vi "Actor Core.vi"(8 "error in":errorcluster, 11 "Nested in":refnum<class "User Interface.lvclass">) -> (0 "error out":errorcluster, 3 "Actor out":refnum<class "Actor.lvclass">)   [LabVIEW 2020, in "User Interface.lvlib" / "User Interface.lvclass"]
doc: "(<B>Filename</B>: Actor Framework.lvlib:Actor.lvclass:Actor Core.vi)\n\nReceives messages to the actor, reacts to them, and initiates any error handling that may shut the actor down.\n\nDescendant classes may override this VI to append parallel tasks for the actor to complete while it handles messages. Overrides use the Call Parent Method node."
uses:
  User Interface.lvclass
  <vilib>/ActorFramework/Actor/Actor.lvclass
  <vilib>/ActorFramework/Stop Msg/Stop Msg.lvclass
  Paquetes Disonibles/Paquetes Disonibles.lvclass
  Manejador de Turnos/Manejador de Turnos.lvclass
  Dinero/Dinero.lvclass
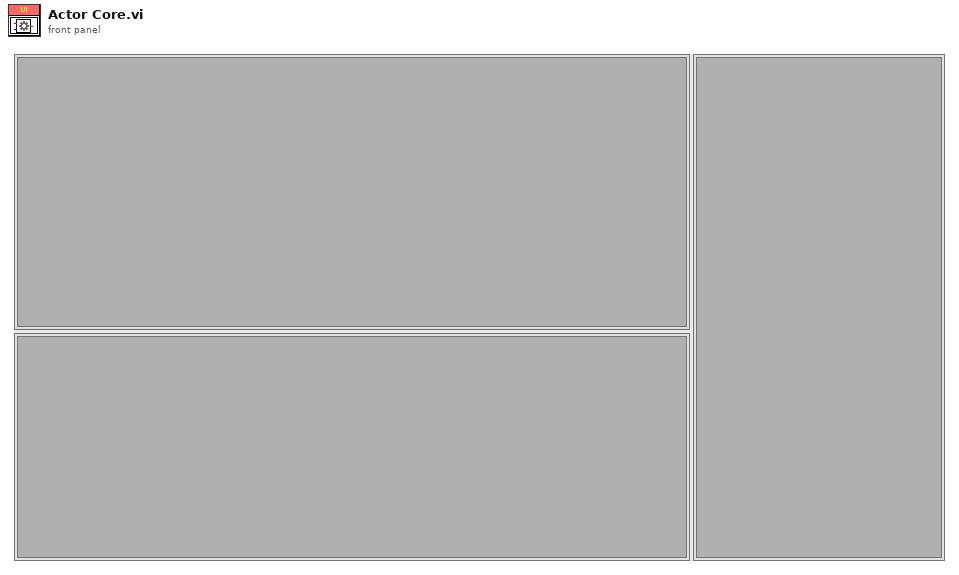
[diagram p1: front panel]
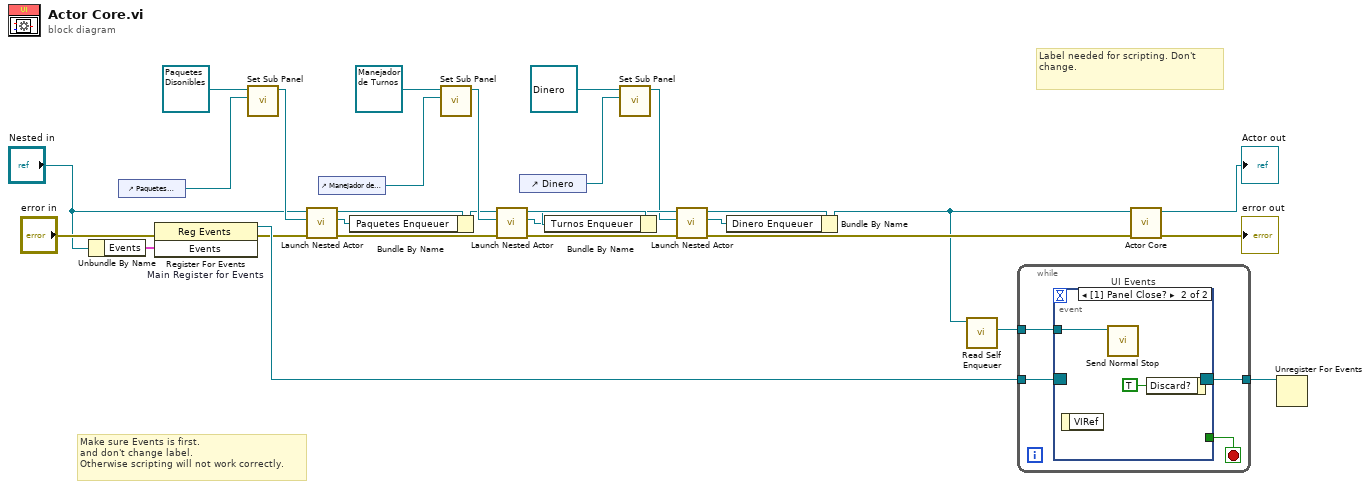
[diagram p0: block diagram]
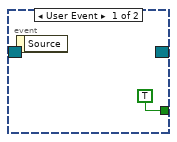
[diagram p2: hidden frame]
diagram:
  # "Label needed for scripting. Don't change."
  # "Make sure Events is first.\nand don't change label.\nOtherwise scripting will not work correctly."
  n1 = Unbundle By Name("Nested in") -> ("Events"=w27:cluster{"Stop":refnum<user-event>})
  n2 = control-ref of="Paquetes disponibles"() -> (w3:refnum<vi>)
  n3 = register-events "Main Register for Events"(error in="error in", w27) -> (reference out=w28:refnum<event-registration>, error out=w19:errorcluster)  [unwired: 1 in]
  n4 = call "Set Sub Panel.vi"("Sub Panel"=w3, "Paquetes Disonibles in"=refnum<class "Paquetes Disonibles.lvclass"> refnum ("Paquetes Disonibles.lvlib:Paquetes Disonibles.lvclass")) -> ("Paquetes Disonibles out"=w18:refnum<class "Paquetes Disonibles.lvclass">)  [unwired: 8 in, 1 out]
  n5 = call <vilib>:"Launch Nested Actor.vi"("error in (no error)"=w19, "Nested Actor"=w18, "Caller Actor in"="Nested in") -> ("error out"=w17:errorcluster, "Nested Actor's Enqueuer"=w4:refnum<class "Message Enqueuer.lvclass">, "Caller Actor out"=w20:refnum<class "User Interface.lvclass">)  [unwired: 6 in]
  n6 = control-ref of="Manejador de turnos"() -> (w2:refnum<vi>)
  n7 = Bundle By Name(cluster=w20, "Paquetes Enqueuer"=w4) -> (w5:refnum<class "User Interface.lvclass">)
  n8 = call "Set Sub Panel.vi"("Sub Panel"=w2, "Manejador de Turnos in"=refnum<class "Manejador de Turnos.lvclass"> refnum ("Manejador de Turnos.lvlib:Manejador de Turnos.lvclass")) -> ("Manejador de Turnos out"=w16:refnum<class "Manejador de Turnos.lvclass">)  [unwired: 8 in, 1 out]
  n9 = call <vilib>:"Launch Nested Actor.vi"("error in (no error)"=w17, "Nested Actor"=w16, "Caller Actor in"=w5) -> ("error out"=w13:errorcluster, "Nested Actor's Enqueuer"=w9:refnum<class "Message Enqueuer.lvclass">, "Caller Actor out"=w14:refnum<class "User Interface.lvclass">)  [unwired: 6 in]
  n10 = control-ref of="Dinero"() -> (w1:refnum<vi>)
  n11 = Bundle By Name(cluster=w14, "Turnos Enqueuer"=w9) -> (w10:refnum<class "User Interface.lvclass">)
  n12 = call "Set Sub Panel.vi"("Sub Panel"=w1, "Dinero in"=refnum<class "Dinero.lvclass"> refnum ("Dinero.lvlib:Dinero.lvclass")) -> ("Dinero out"=w8:refnum<class "Dinero.lvclass">)  [unwired: 8 in, 1 out]
  n13 = call <vilib>:"Launch Nested Actor.vi"("error in (no error)"=w13, "Nested Actor"=w8, "Caller Actor in"=w10) -> ("error out"=w12:errorcluster, "Nested Actor's Enqueuer"=w6:refnum<class "Message Enqueuer.lvclass">, "Caller Actor out"=w11:refnum<class "User Interface.lvclass">)  [unwired: 6 in]
  n14 = Bundle By Name(cluster=w11, "Dinero Enqueuer"=w6) -> (w7:refnum<class "User Interface.lvclass">)
  n15 = call <vilib>:"Read Self Enqueuer.vi"("Actor"=w7) -> ("Self Enqueuer"=w25:refnum<class "Message Enqueuer.lvclass">)  [unwired: 10 in]
  n16 = while {
    tunnel: w28 -> [w34]
    tunnel: [w32] -> w26
    tunnel: w25 -> [w31]
    stop <- w33 stop-if-true
    n17 = event "UI Events" shown="[1] Panel Close?" {
      selector: w34 -> [_ _]
      dyn-events: [_ _] -> w32
      timeout: _ -> [_ _]
      tunnel: [TRUE _] -> w33
      tunnel: w31 -> [_ w36]
      event User Event {
        n18 = event-data() -> ()  [unwired: 1 in, 1 out]
      }
      event Panel Close? {
        n19 = event-data() -> ()  [unwired: 1 in, 1 out]
        n20 = call <vilib>:"Send Normal Stop.vi"("Message Enqueuer"=w36) -> ()  [unwired: 10 in, 1 out]
        n21 = event-data("Discard?"=TRUE) -> ()  [unwired: 1 in, 1 out]
      }
    }
  }
  n22 = call-parent "Actor Core.vi"("error in"=w12, "Actor in"=w7) -> ("error out"=→"error out":errorcluster, "Actor out"=→"Actor out":refnum<class "Actor.lvclass">)  [unwired: 8 in]
  n23 = Unregister For Events(event registration refnum=w26) -> ()  [unwired: 1 in, 1 out]
